vi "压力.vi"(9 "Bool引用句柄":refnum<vi>, 10 "簇":T4, 11 "事件注册引用句柄 2":refnum<event-registration>) -> ()   [LabVIEW 2020]
uses:
  <vilib>/Utility/miscctls.llb/LVRowAndColumnUnsignedTypeDef.ctl
  <vilib>/Utility/miscctls.llb/LVRectTypeDef.ctl
  Windows/System32/user32.dll
panel:
  in  "布尔 3":T1
  in  "布尔 2":T2
  in  "布尔":T3
  out "数值":dbl format="%#_2f Pa"
  in  "表格":string[][](table)
  out "波形图":dbl[](graph)
  # "压力数据"
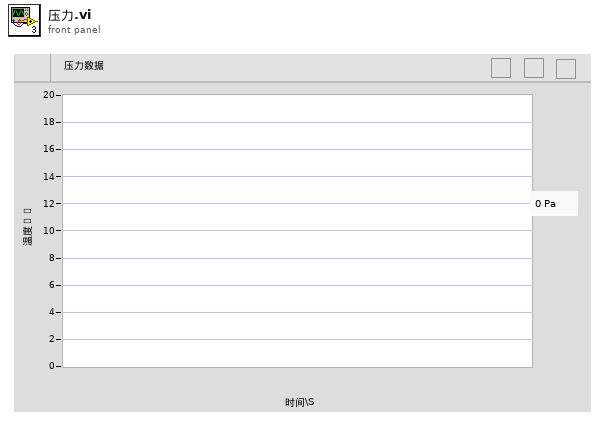
[diagram p1: front panel]
types:
  T1 = typedef "控件关闭.ctl" = bool
  T2 = typedef "控件最小化.ctl" = bool
  T3 = typedef "控件最大化.ctl" = bool
  T4 = cluster{"A1温度":refnum<vi>, "A2温度":refnum<vi>, "A3温度":refnum<vi>, "A4温度":refnum<vi>}
  T5 = typedef "LVRectTypeDef.ctl" = cluster{"Left":i16, "Top":i16, "Right":i16, "Bottom":i16}
  T6 = typedef "LVRowAndColumnUnsignedTypeDef.ctl" = cluster{"Row":u32, "Column":u32}
  T7 = typedef "LVPoint32TypeDef.ctl" = cluster{"Horizontal":i32, "Vertical":i32}
  T8 = enum32{"Invalid", "Standard", "Closed", "Hidden", "Minimized", "Maximized"}
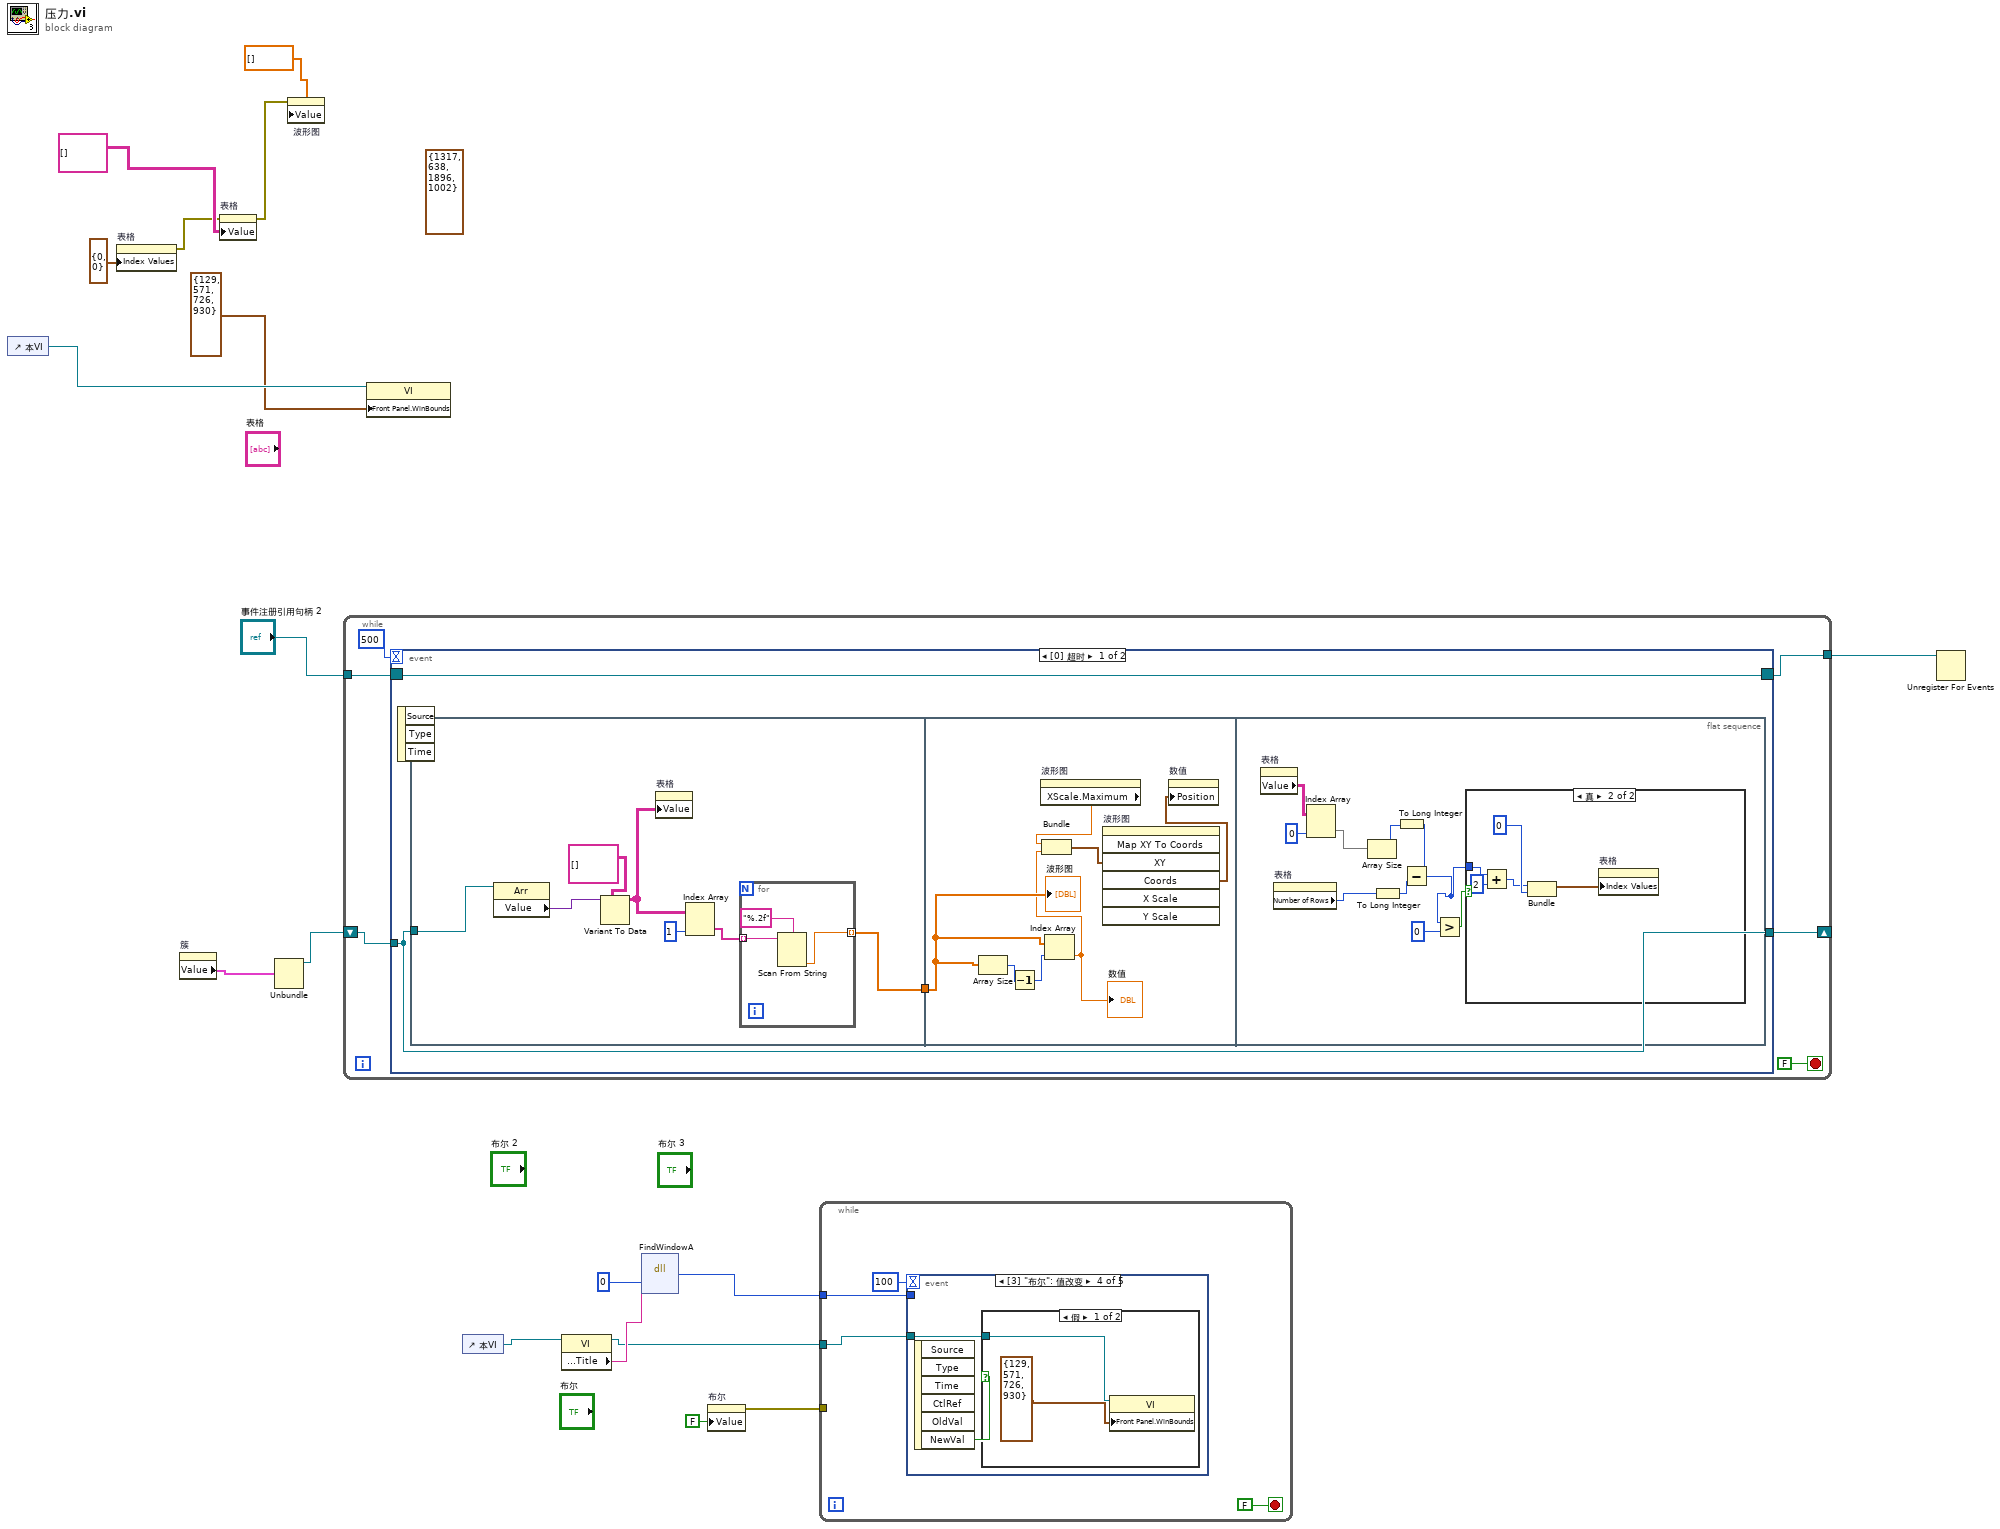
[diagram p0: block diagram]
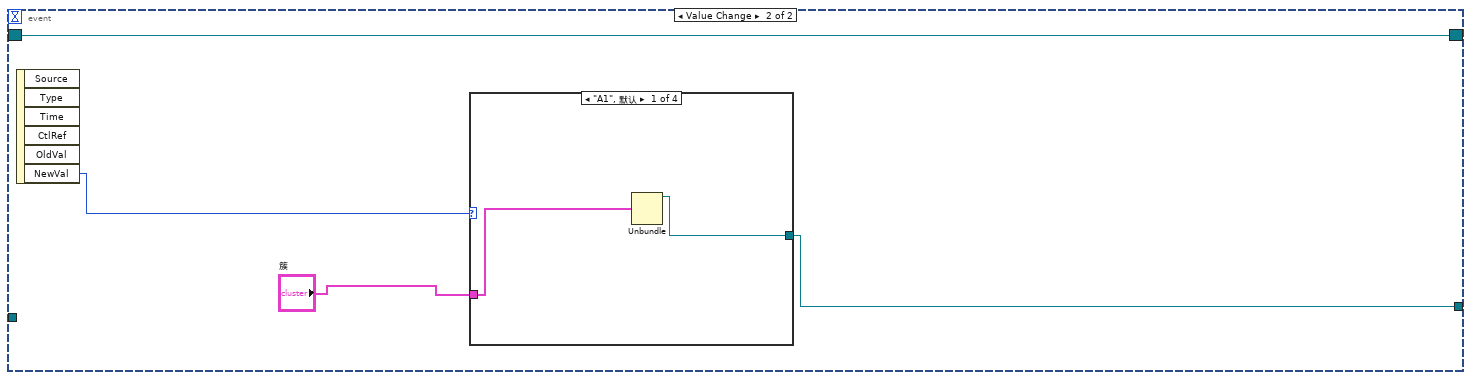
[diagram p3: hidden frame]
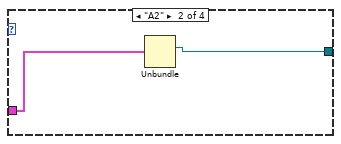
[diagram p4: hidden frame]
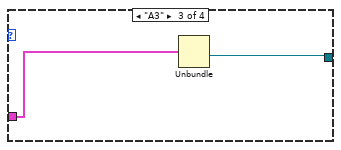
[diagram p5: hidden frame]
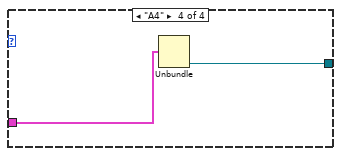
[diagram p6: hidden frame]
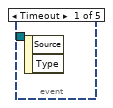
[diagram p7: hidden frame]
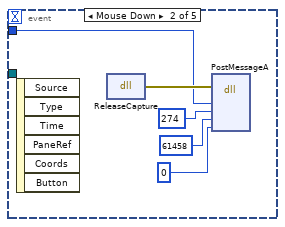
[diagram p8: hidden frame]
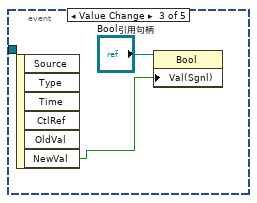
[diagram p9: hidden frame]
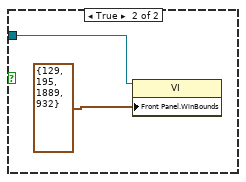
[diagram p10: hidden frame]
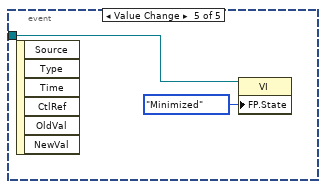
[diagram p11: hidden frame]
diagram:
  (unwired) T5 {"Left"=1317, "Top"=638, "Right"=1896, "Bottom"=1002} ("前面板窗口:窗口边界")
  n1 = control-ref of="本VI"() -> (w7:refnum<vi>)
  n2 = property on="表格" class="Tbl (严格)"("Index Values"=T6 {"Row"=0, "Column"=0} ("索引值")) -> (error out=w9:errorcluster)  [unwired: 2 in, 1 out]
  n3 = property on="簇" class="Clust (严格)"() -> ("Value"=w5:T4)  [unwired: 2 in, 2 out]
  n4 = property on="表格" class="Tbl (严格)"(error in=w9, "Value"=string[][] []) -> (error out=w10:errorcluster)  [unwired: 1 in, 1 out]
  n5 = Unbundle(w5) -> ("A1温度"=w4:refnum<vi>)  [unwired: 3 out]
  n6 = property on="波形图" class="WFGraph (严格)"(error in=w10, "Value"=dbl[] []) -> ()  [unwired: 1 in, 2 out]
  n7 = while {
    tunnel: "事件注册引用句柄 2" -> [w23]
    shift-right: [w21] -> _
    shift-left: w4 -> [w22]
    tunnel: [w20] -> w3
    stop <- FALSE stop-if-true
    n8 = event shown="[0] 超时" {
      selector: w23 -> [w26 w60]
      dyn-events: [w26 w60] -> w20
      timeout: 500 -> [_ _]
      tunnel: w22 -> [w25 _]
      tunnel: [w25 w61] -> w21
      event Timeout {
        n9 = event-data() -> ()  [unwired: 1 in, 3 out]
        n10 = flat-sequence {
          tunnel: [w30] -> w27
          tunnel: w25 -> [w29]
          tunnel: w27 -> [w40]
          frame #0 {
            n11 = property class="Arr"(reference=w29) -> ("Value"=w34:variant)  [unwired: 1 in, 2 out]
            n12 = Variant To Data(type=string[][] [], Variant=w34) -> (data=w28:string[][])  [unwired: 1 in, 1 out]
            n13 = property on="表格" class="Tbl (严格)"("Value"=w28) -> ()  [unwired: 2 in, 2 out]
            n14 = Index Array(array=w28, index (col)=1 ("禁用的索引 (列)")) -> (element=w31:string[])  [unwired: 1 in]
            n15 = for {
              tunnel: w31 -> [w37] mode=indexing
              tunnel: [w35] -> w30 mode=indexing
              n16 = Scan From String(format string="%.2f" ("格式字符串"), input string=w37) -> (output 1=w35:dbl)  [unwired: 3 in, 3 out]
            }
          }
          frame #1 {
            n17 = Array Size(array=w40) -> (size(s)=w42:i32)
            n18 = Decrement(x=w42) -> (x-1=w41:i32)
            n19 = property on="波形图" class="WFGraph (严格)"() -> ("XScale.Maximum"=w43:dbl)  [unwired: 2 in, 2 out]
            n20 = Index Array(array=w40, index=w41) -> (element=w39:dbl)
            "数值" <- w39
            n21 = Bundle("XScale.Maximum"=w43, w39) -> (w38:cluster{"XScale.Maximum":dbl, dbl})  [unwired: 1 in]
            n22 = invoke on="波形图" class="WFGraph (严格)" method="Map XY To Coords"("XY"=w38) -> ("Coords"=w44:T7)  [unwired: 6 in, 6 out]
            n23 = property on="数值" class="DigNum (严格)"("Position"=w44) -> ()  [unwired: 2 in, 2 out]
            "波形图" <- w40
          }
          frame #2 {
            n24 = property on="表格" class="Tbl (严格)"() -> ("Value"=w54:string[][])  [unwired: 2 in, 2 out]
            n25 = property on="表格" class="Tbl (严格)"() -> ("Number of Rows"=w48:u32)  [unwired: 2 in, 2 out]
            n26 = Index Array(array=w54, index (col)=0 ("禁用的索引 (列)")) -> (element=w52:string[])  [unwired: 1 in]
            n27 = Array Size(array=w52) -> (size(s)=w50:i32)
            n28 = To Long Integer(number=w48) -> (32bit integer=w47:i32)
            n29 = To Long Integer(number=w50) -> (32bit integer=w49:i32)
            n30 = Subtract(x=w49, y=w47) -> (x-y=w45:i32)
            n31 = Greater?(x=w45, y=0) -> (0:w51:bool)
            n32 = case shown="真" w51 {
              tunnel: w45 -> [_ w57]
              frame False {
              }
              frame True {
                n33 = Add(x=w57, y=2) -> (x+y=w55:i32)
                n34 = Bundle(w55, 0) -> (w59:cluster{i32, i32})  [unwired: 1 in]
                n35 = property on="表格" class="Tbl (严格)"("Index Values"=w59) -> ()  [unwired: 2 in, 2 out]
              }
            }
          }
        }
      }
      event Value Change {
        n36 = event-data() -> ("NewVal"=w63:enum32{"未选择", "A1", "A2", "A3", "A4"})  [unwired: 1 in, 5 out]
        n37 = case shown="\"A1\", 默认" w63 {
          tunnel: "簇" -> [w64 w67 w69 w71]
          tunnel: [w65 w66 w68 w70] -> w61
          frame "A1", Default {
            n38 = Unbundle(w64) -> ("A1温度"=w65:refnum<vi>)  [unwired: 3 out]
          }
          frame "A2" {
            n39 = Unbundle(w67) -> ("A2温度"=w66:refnum<vi>)  [unwired: 3 out]
          }
          frame "A3" {
            n40 = Unbundle(w69) -> ("A3温度"=w68:refnum<vi>)  [unwired: 3 out]
          }
          frame "A4" {
            n41 = Unbundle(w71) -> ("A4温度"=w70:refnum<vi>)  [unwired: 3 out]
          }
        }
      }
    }
  }
  n42 = property class="VI"(reference=w7, "Front Panel.WinBounds"=T5 {"Left"=129, "Top"=571, "Right"=726, "Bottom"=930} ("前面板窗口:前面板边界")) -> ()  [unwired: 1 in, 2 out]
  n43 = control-ref of="本VI"() -> (w17:refnum<vi>)
  n44 = property class="VI"(reference=w17) -> (reference out=w12:refnum<vi>, "Front Panel.Title"=w16:string)  [unwired: 1 in, 1 out]
  n45 = dll-call lib="/Windows/System32/user32.dll" fn="FindWindowA"("lp"=u32 0, "name"=w16) -> ("返回类型"=w15:u32)  [unwired: 5 in, 2 out]
  n46 = property on="布尔" class="Bool (严格)"("Value"=T3 FALSE ("布尔")) -> (error out=w13:errorcluster)  [unwired: 2 in, 1 out]
  n47 = while {
    tunnel: w15 -> [w75]
    tunnel: w13 -> [_]
    tunnel: w12 -> [w74]
    stop <- FALSE stop-if-true
    n48 = event shown="[3] \"布尔\": 值改变" {
      selector: _ -> [_ _ _ _ _]
      dyn-events: _ -> [_ _ _ _ _]
      timeout: 100 -> [_ _ _ _ _]
      tunnel: w75 -> [_ w79 _ _ _]
      tunnel: w74 -> [_ _ _ w83 w90]
      event Timeout {
        n49 = event-data() -> ()  [unwired: 1 in, 2 out]
      }
      event Mouse Down {
        n50 = event-data() -> ()  [unwired: 1 in, 6 out]
        n51 = dll-call lib="/Windows/System32/user32.dll" fn="ReleaseCapture"() -> (error out=w80:errorcluster)  [unwired: 4 in, 1 out]
        n52 = dll-call lib="/Windows/System32/user32.dll" fn="PostMessageA"(error in=w80, "lp"=w79, "name"=274, "vak"=61458, "val"=0) -> ()  [unwired: 7 in, 2 out]
      }
      event Value Change {
        n53 = event-data() -> ("NewVal"=w81:T1)  [unwired: 1 in, 5 out]
        n54 = property class="Bool"(reference="Bool引用句柄", "Val(Sgnl)"=w81) -> ()  [unwired: 1 in, 2 out]
      }
      event Value Change {
        n55 = event-data() -> ("NewVal"=w84:T3)  [unwired: 1 in, 5 out]
        n56 = case shown="假" w84 {
          tunnel: w83 -> [w86 w87]
          frame False {
            n57 = property class="VI"(reference=w86, "Front Panel.WinBounds"=T5 {"Left"=129, "Top"=571, "Right"=726, "Bottom"=930} ("前面板窗口:前面板边界")) -> ()  [unwired: 1 in, 2 out]
          }
          frame True {
            n58 = property class="VI"(reference=w87, "Front Panel.WinBounds"=T5 {"Left"=129, "Top"=195, "Right"=1889, "Bottom"=932} ("前面板窗口:前面板边界")) -> ()  [unwired: 1 in, 2 out]
          }
        }
      }
      event Value Change {
        n59 = event-data() -> ()  [unwired: 1 in, 6 out]
        n60 = property class="VI"(reference=w90, "FP.State"=T8."Minimized" ("前面板窗口:状态")) -> ()  [unwired: 1 in, 2 out]
      }
    }
  }
  n61 = Unregister For Events(event registration refnum=w3) -> ()  [unwired: 1 in, 1 out]
